vi "Log Command Message.vi"(6 "Command Message":refnum<class "Command Message Interface.lvclass">, 7 "Actor":refnum<class "Ancestral Actor.lvclass">, 8 "error in (no error)":errorcluster, 11 "Level":T1) -> (0 "error out":errorcluster)   [LabVIEW 2016, in "Stream Log.lvlib" / "Global Application Log.lvclass"]
doc: "--\nCopyright © 2017 Composed SystemsI All rights reserved.\n\nAuthor: Jon McBee <jon.mcbee@composed.io>\n\nThis library is provided \"AS IS\" ,WITHOUT WARRANTIES OR\nCONDITIONS OF ANY KIND, either express or implied.\n\nComposed Systems -- composed.io\n\nStream 0.0.1.1\nJon McBee - Composed Systems\nCopyright (c) 2017, Composed Systems"
uses:
  <userlib>/Composed Systems/Stream/Log/Global Application Log/Global Application Log.lvclass
  <userlib>/Composed Systems/Stream/Log/Application Log/Log Level.ctl
  <userlib>/Composed Systems/Stream/Mediator/Classes/Message Command Interface/Command Message Interface.lvclass
  <userlib>/Composed Systems/Stream/Actor/Actor Class/Ancestral Actor.lvclass
  <userlib>/Composed Systems/Stream/Log/Global Application Log/Global Application Log.lvclass/Global Application Log.ctl
  <userlib>/Composed Systems/Stream/Log/Application Log/Application Log.lvclass
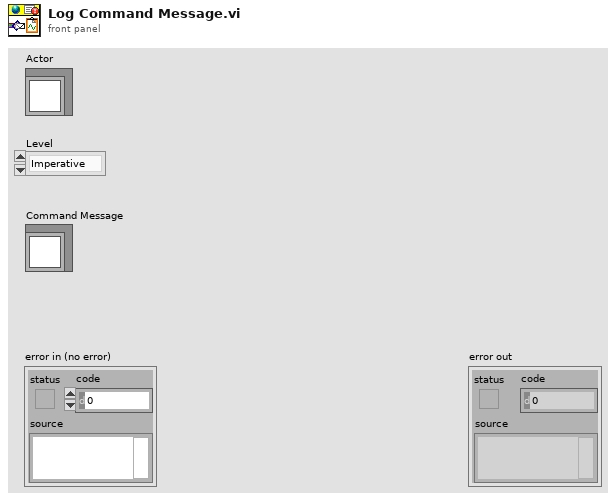
[diagram p1: front panel]
types:
  T1 = typedef "Stream Log.lvlib/Application Log.lvclass/Log Level.ctl" = enum16{"Imperative", "Major", "Minor", "Debug", "Off"}
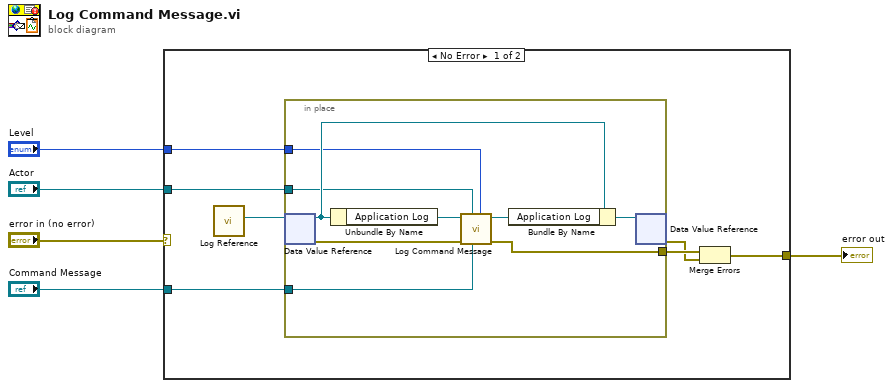
[diagram p0: block diagram]
diagram:
  n1 = case shown="No Error" "error in (no error)" {
    selector: "error in (no error)" -> [_ w22]
    tunnel: [w9 w22] -> w4
    tunnel: "Level" -> [w8 _]
    tunnel: "Actor" -> [w7 _]
    tunnel: "Command Message" -> [w6 _]
    frame No Error {
      n2 = call <userlib>:"Log Reference.vi"() -> ("Global Log Reference out"=w12:refnum<data-value>)  [unwired: 11 in]
      n3 = in-place {
        in-place-border: [w18] -> w11
        in-place-border: w8 -> [w17]
        in-place-border: w7 -> [w14]
        in-place-border: w6 -> [w13]
        n4 = in-place-dvr #1(w12) -> (w21:refnum<class "Global Application Log.lvclass">, w19:errorcluster)
        n5 = Unbundle By Name(w21) -> ("Application Log"=w15:refnum<class "Application Log.lvclass">)
        n6 = call <userlib>:"Log Command Message.vi"("Level"=w17, "Command Message"=w13, "Actor"=w14, "error in (no error)"=w19, "Application Log in"=w15) -> ("error out"=w18:errorcluster, "Application Log out"=w16:refnum<class "Application Log.lvclass">)  [unwired: 5 in]
        n7 = Bundle By Name(cluster=w21, "Application Log"=w16) -> (w20:refnum<class "Global Application Log.lvclass">)
        n8 = in-place-dvr #1(w20) -> (w10:errorcluster)  [unwired: 1 out]
      }
      n9 = Merge Errors(w11, w10) -> (w9:errorcluster)
    }
    frame Error {
    }
  }
  "error out" <- w4
